vi "Untitled 1.vi"() -> ()   [LabVIEW 2017]
panel:
  out "error out":errorcluster
  out "return count":u32
  out "find list":string[](array[string])
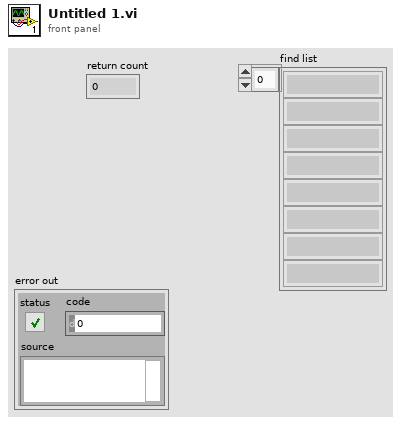
[diagram p1: front panel]
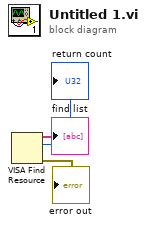
[diagram p0: block diagram]
diagram:
  n1 = VISA Find Resource() -> (0:→"error out":errorcluster, 2:→"return count":u32, 3:→"find list":string[])  [unwired: 3 in]
